vi "XYROI.vi"(4 "y-":i32, 6 "y+":i32, 7 "X+":i32, 9 "Y raw":i32[](array[numeric]), 10 "X raw":i32[](array[numeric]), 11 "X-":i32) -> (1 "XY ROI":cluster{i32[], i32[]}, 2 "Y in ROI":i32[](array[numeric]), 3 "X in ROI":i32[](array[numeric]))   [LabVIEW 2021]
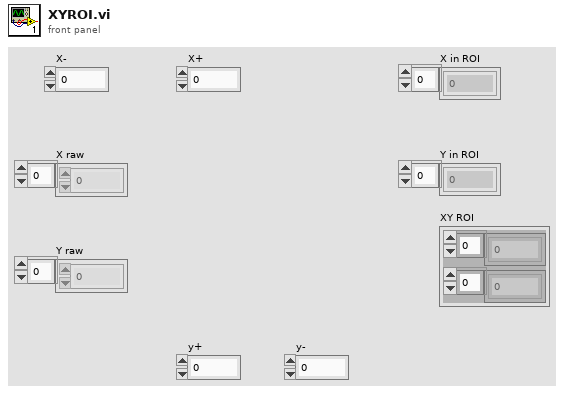
[diagram p1: front panel]
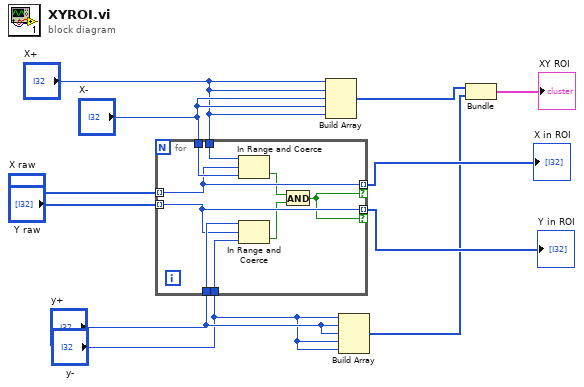
[diagram p0: block diagram]
diagram:
  n1 = for {
    tunnel: "X raw" -> [w16] mode=indexing
    tunnel: "Y raw" -> [w15] mode=indexing
    tunnel: "X+" -> [w20]
    tunnel: "X-" -> [w19]
    tunnel: "y+" -> [w18]
    tunnel: "y-" -> [w17]
    tunnel: [w16] -> w10 mode=indexing if=w12
    tunnel: [w15] -> w11 mode=indexing if=w12
    n2 = In Range and Coerce(upper limit=w20, x=w16, lower limit=w19) -> (In Range?=w14:bool)  [unwired: 1 out]
    n3 = In Range and Coerce(upper limit=w18, x=w15, lower limit=w17) -> (In Range?=w13:bool)  [unwired: 1 out]
    n4 = And(x=w14, y=w13) -> (x .and. y?=w12:bool)
  }
  "Y in ROI" <- w11
  "X in ROI" <- w10
  n5 = Build Array("X+", "X+", "X-", "X-", "X+") -> (w3:i32[])
  n6 = Build Array("y-", "y+", "y+", "y-", "y-") -> (w2:i32[])
  n7 = Bundle(w3, w2) -> (→"XY ROI":cluster{i32[], i32[]})  [unwired: 1 in]
